vi "ConfigureChannels.vi"(6 "supported metrics":string[](array[string]), 7 "high rate":bool, 8 "error in (no error)":errorcluster, 9 "metric cache":variant, 10 "group":T1, 11 "device":T10) -> (0 "error out":errorcluster, 2 "valid config":bool, 3 "channels":T6[](array[typedef]))   [LabVIEW 2017, in "AnalysisHelper.lvlib"]
uses:
  <vilib>/addons/InsightCM/Utilities/Analysis/Shared/AnalysisHelper.lvlib
  <vilib>/addons/InsightCM/MessageBus/Base/controls/R2_DeviceModel.ctl
  <vilib>/addons/InsightCM/MessageBus/Base/controls/R2_Device.ctl
  <vilib>/addons/InsightCM/MessageBus/Base/controls/KeyValuePair.ctl
  <vilib>/addons/InsightCM/MessageBus/Base/controls/DeviceState.ctl
  <vilib>/addons/InsightCM/MessageBus/Base/controls/R2_DataGroup.ctl
  <vilib>/addons/InsightCM/MessageBus/Base/controls/OperatingState.ctl
  <vilib>/addons/InsightCM/MessageBus/Base/controls/Trigger.ctl
  <vilib>/addons/InsightCM/MessageBus/Base/controls/Condition.ctl
  <vilib>/addons/InsightCM/MessageBus/Base/controls/BurstModeTrigger.ctl
  <vilib>/addons/InsightCM/MessageBus/Base/controls/DeviceSensorGroup.ctl
  <vilib>/addons/InsightCM/MessageBus/Base/controls/WirelessEndpoint.ctl
  <vilib>/addons/InsightCM/MessageBus/Base/controls/WirelessChannel.ctl
  <vilib>/addons/InsightCM/MessageBus/Base/controls/R2_Channel.ctl
  <vilib>/addons/InsightCM/MessageBus/Base/controls/Metric.ctl
  <vilib>/addons/InsightCM/MessageBus/Base/controls/Tag.ctl
  <vilib>/addons/InsightCM/Utilities/Analysis/Shared/controls/Channel.ctl
  <vilib>/addons/InsightCM/Utilities/Analysis/Shared/controls/SpeedType.ctl
  <vilib>/addons/InsightCM/Utilities/Analysis/Shared/controls/Feature.ctl
  <vilib>/addons/InsightCM/Utilities/Analysis/Shared/controls/AmplitudeScale.ctl
  <vilib>/addons/InsightCM/Utilities/Analysis/Shared/controls/SpeedCacheOps.ctl
  <vilib>/addons/InsightCM/Utilities/DeviceModelHelpers/DeviceModelHelpers.lvlib
  <vilib>/addons/InsightCM/Utilities/PropertyHelpers/PropertyHelpers.lvlib
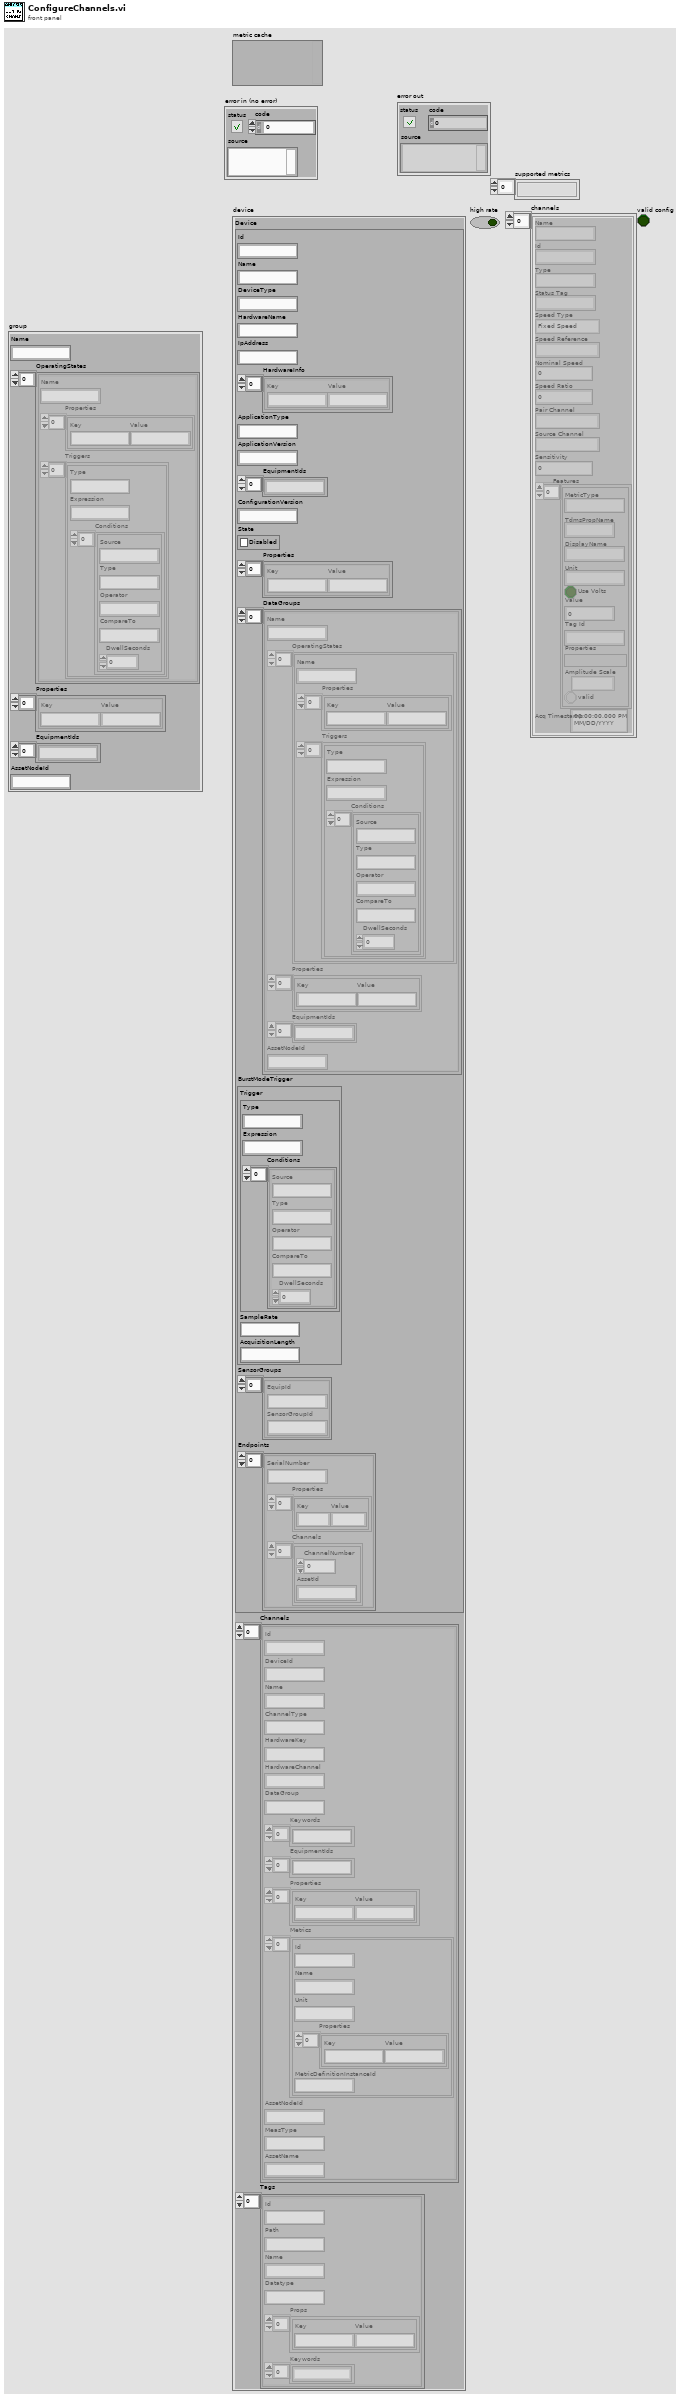
[diagram p1: front panel]
types:
  T1 = typedef "R2_DataGroup.ctl" = cluster{"Name":string, "OperatingStates":T2[], "Properties":T3[], "EquipmentIds":string[], "AssetNodeId":string}
  T2 = typedef "OperatingState.ctl" = cluster{"Name":string, "Properties":T3[], "Triggers":T4[]}
  T3 = typedef "KeyValuePair.ctl" = cluster{"Key":string, "Value":string}
  T4 = typedef "Trigger.ctl" = cluster{"Type":string, "Expression":string, "Conditions":T5[]}
  T5 = typedef "Condition.ctl" = cluster{"Source":string, "Type":string, "Operator":string, "CompareTo":string, "DwellSeconds":dbl}
  T6 = typedef "AnalysisHelper.lvlib/Channel.ctl" = cluster{"Name":string, "Id":string, "Type":string, "Status Tag":string, "Speed Type":T7, "Speed Reference":string, "Nominal Speed":dbl, "Speed Ratio":dbl, "Pair Channel":string, "Source Channel":string, "Sensitivity":dbl, "Features":T8[], "Acq Timestamp":timestamp}
  T7 = typedef "AnalysisHelper.lvlib/SpeedType.ctl" = enum16{"Fixed Speed", "Tachometer", "From Map"}
  T8 = typedef "AnalysisHelper.lvlib/Feature.ctl" = cluster{"MetricType":string, "TdmsPropName":string, "DisplayName":string, "Unit":string, "Use Volts":bool, "Value":dbl, "Tag Id":string, "Properties":variant, "Amplitude Scale":T9, "valid":bool}
  T9 = typedef "AnalysisHelper.lvlib/AmplitudeScale.ctl" = enum16{"rms", "peak", "pk-pk"}
  T10 = typedef "R2_DeviceModel.ctl" = cluster{"Device":T11, "Channels":T17[], "Tags":T19[]}
  T11 = typedef "R2_Device.ctl" = cluster{"Id":string, "Name":string, "DeviceType":string, "HardwareName":string, "IpAddress":string, "HardwareInfo":T3[], "ApplicationType":string, "ApplicationVersion":string, "EquipmentIds":string[], "ConfigurationVersion":string, "State":T12, "Properties":T3[], "DataGroups":T1[], "BurstModeTrigger":T13, "SensorGroups":T14[], "Endpoints":T15[]}
  T12 = typedef "DeviceState.ctl" = cluster{"Disabled":bool}
  T13 = typedef "BurstModeTrigger.ctl" = cluster{"Trigger":T4, "SampleRate":string, "AcquisitionLength":string}
  T14 = typedef "DeviceSensorGroup.ctl" = cluster{"EquipId":string, "SensorGroupId":string}
  T15 = typedef "WirelessEndpoint.ctl" = cluster{"SerialNumber":string, "Properties":T3[], "Channels":T16[]}
  T16 = typedef "WirelessChannel.ctl" = cluster{"ChannelNumber":i32, "AssetId":string}
  T17 = typedef "R2_Channel.ctl" = cluster{"Id":string, "DeviceId":string, "Name":string, "ChannelType":string, "HardwareKey":string, "HardwareChannel":string, "DataGroup":string, "Keywords":string[], "EquipmentIds":string[], "Properties":T3[], "Metrics":T18[], "AssetNodeId":string, "MeasType":string, "AssetName":string}
  T18 = typedef "Metric.ctl" = cluster{"Id":string, "Name":string, "Unit":string, "Properties":T3[], "MetricDefinitionInstanceId":string}
  T19 = typedef "Tag.ctl" = cluster{"Id":string, "Path":string, "Name":string, "Datatype":string, "Props":T3[], "Keywords":string[]}
  T20 = typedef "AnalysisHelper.lvlib/SpeedCacheOps.ctl" = enum16{"Init", "GetSpeed"}
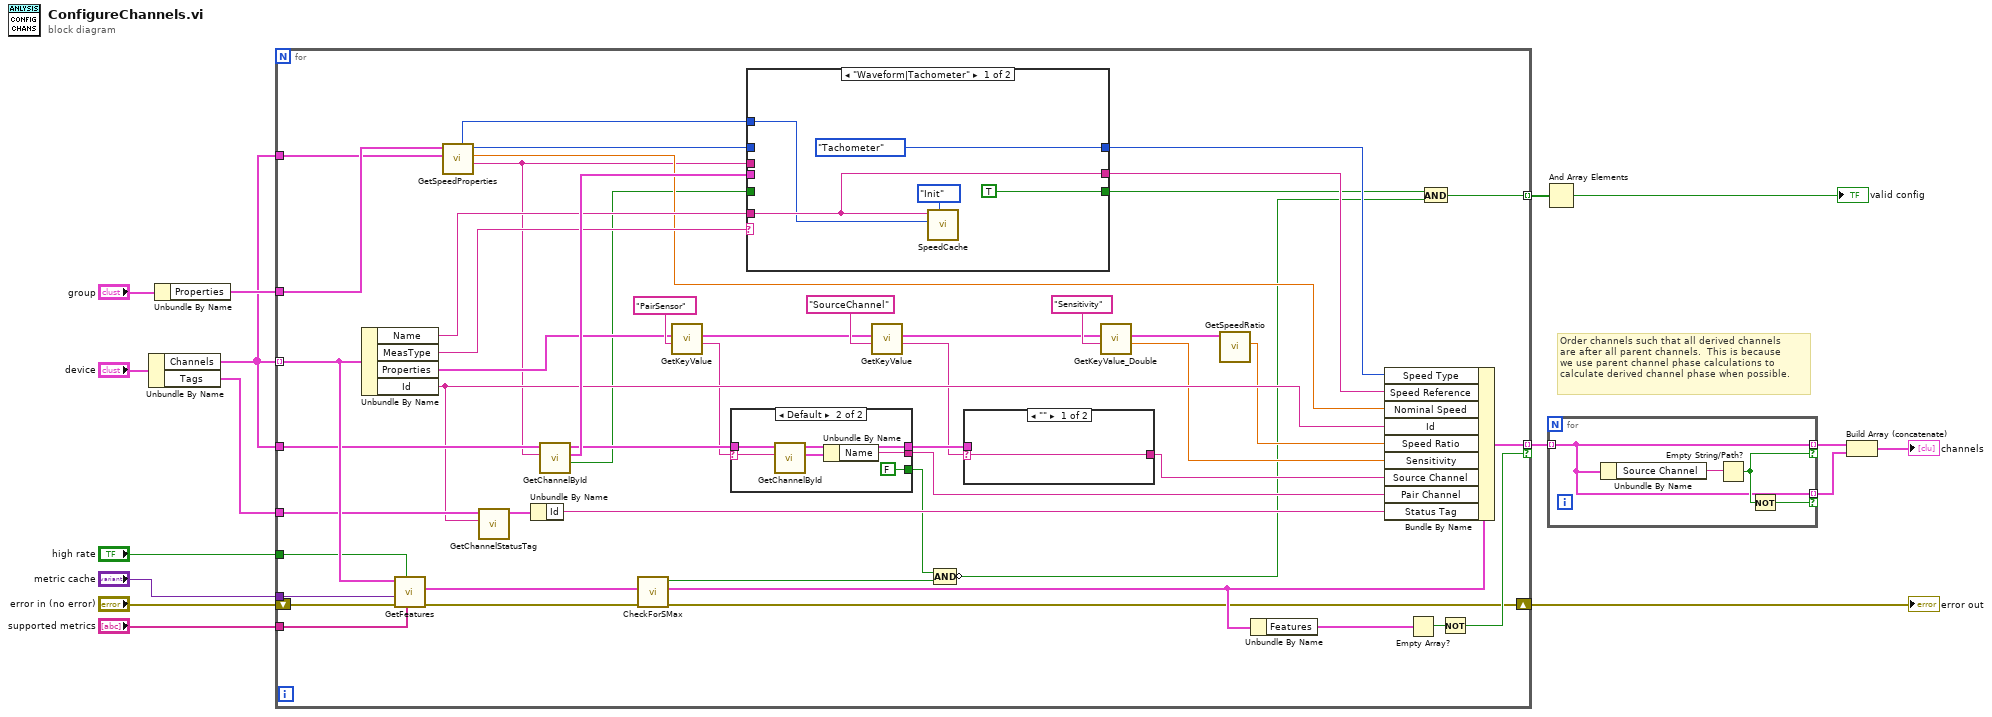
[diagram p0: block diagram]
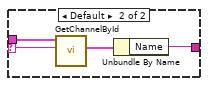
[diagram p2: hidden frame]
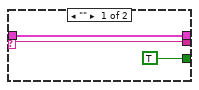
[diagram p3: hidden frame]
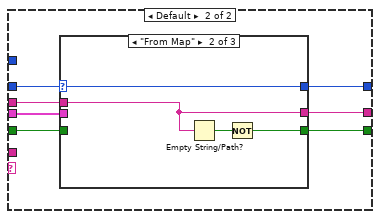
[diagram p4: hidden frame]
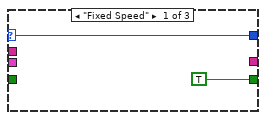
[diagram p5: hidden frame]
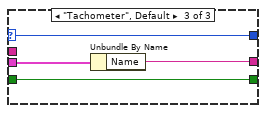
[diagram p6: hidden frame]
diagram:
  # "Order channels such that all derived channels\nare after all parent channels.  This is because\nwe use parent channel phase calculations to\ncalculate derived channel phase when possible."
  n1 = Unbundle By Name("device") -> ("Channels"=w1:T17[], "Tags"=w13:T19[])
  n2 = Unbundle By Name("group") -> ("Properties"=w11:T3[])
  n3 = for {
    tunnel: [w63] -> w9 mode=indexing if=w45
    tunnel: "metric cache" -> [w65]
    tunnel: w1 -> [w64] mode=indexing
    tunnel: w13 -> [w51]
    shift-right: [w27] -> w10
    shift-left: "error in (no error)" -> [w66]
    tunnel: w1 -> [w60]
    tunnel: w11 -> [w42]
    tunnel: "supported metrics" -> [w48]
    tunnel: "high rate" -> [w30]
    tunnel: [w21] -> w3 mode=indexing
    tunnel: w1 -> [w18]
    n4 = Unbundle By Name(w64) -> ("Name"=w58:string, "MeasType"=w57:string, "Properties"=w40:T3[], "Id"=w43:string)
    n5 = call <vilib>:"GetFeatures.vi"("supported metrics"=w48, "high rate"=w30, "error in (no error)"=w66, "Metric Cache"=w65, "ChannelModel"=w64) -> ("error out"=w28:errorcluster, "Chanel"=w26:T6)  [unwired: 5 in]
    n6 = call <vilib>:"GetSpeedProperties.vi"("Channels"=w18, "properties"=w42) -> ("speed reference id"=w19:string, "nominal speed"=w41:dbl, "speed type"=w39:T7, "max empty blocks"=w17:i32)  [unwired: 6 in]
    n7 = call <vilib>:"GetChannelStatusTag.vi"("channel id"=w43, "tags"=w51) -> ("channel status tag"=w50:T19)  [unwired: 9 in]
    n8 = Unbundle By Name(w50) -> ("Id"=w49:string)
    n9 = call <vilib>:"GetChannelById.vi"("channel id"=w19, "channels in"=w60) -> ("found"=w23:bool, "channel"=w62:T17, "channels out"=w61:T17[])  [unwired: 7 in]
    n10 = call <vilib>:"CheckForSMax.vi"("error in (no error)"=w28, "chanel in"=w26) -> ("error out"=w27:errorcluster, "chanel out"=w29:T6, "contains smax"=w25:bool)  [unwired: 7 in]
    n11 = call <vilib>:"GetKeyValue.vi"("key"="PairSensor", "key value pairs"=w40) -> ("value"=w36:string, "key value pairs out"=w44:T3[])  [unwired: 7 in, 1 out]
    n12 = case shown="Default" w36 {
      selector: w36 -> [w73 w76]
      tunnel: w61 -> [w74 w79]
      tunnel: [w73 w78] -> w59
      tunnel: [w74 w77] -> w52
      tunnel: [TRUE FALSE] -> w24
      frame "" {
      }
      frame Default {
        n13 = call <vilib>:"GetChannelById.vi"("channel id"=w76, "channels in"=w79) -> ("channel"=w80:T17, "channels out"=w77:T17[])  [unwired: 7 in, 1 out]
        n14 = Unbundle By Name(w80) -> ("Name"=w78:string)
      }
    }
    n15 = case shown="\"Waveform|Tachometer\"" w57 {
      tunnel: w62 -> [_ w92]
      tunnel: w58 -> [w84 _]
      tunnel: [w84 w91] -> w38
      tunnel: [SpeedType."Tachometer" ("speed type") w89] -> w37
      tunnel: w39 -> [_ w90]
      tunnel: w23 -> [_ w88]
      tunnel: [TRUE ("found") w87] -> w20
      tunnel: w19 -> [_ w86]
      tunnel: w17 -> [w81 _]
      frame "Waveform|Tachometer" {
        n16 = call <vilib>:"SpeedCache.vi"("operation"=SpeedCacheOps."Init", "max empty blocks"=w81, "channel"=w84) -> ()  [unwired: 6 in, 3 out]
      }
      frame Default {
        n17 = case shown="\"From Map\"" w90 {
          selector: w90 -> [w94 w98 w100]
          tunnel: w92 -> [_ _ w102]
          tunnel: [_ w97 w101] -> w91
          tunnel: [w94 w98 w100] -> w89
          tunnel: w88 -> [_ _ w99]
          tunnel: [TRUE ("found") w95 w99] -> w87
          tunnel: w86 -> [_ w97 _]
          frame "Fixed Speed" {
          }
          frame "From Map" {
            n18 = Empty String/Path?(string/path=w97) -> (empty?=w96:bool)
            n19 = Not(x=w96) -> (.not. x?=w95:bool)
          }
          frame "Tachometer", Default {
            n20 = Unbundle By Name(w102) -> ("Name"=w101:string)
          }
        }
      }
    }
    n21 = call <vilib>:"GetKeyValue.vi"("key"="SourceChannel", "key value pairs"=w44) -> ("value"=w35:string, "key value pairs out"=w34:T3[])  [unwired: 7 in, 1 out]
    n22 = Compound Arithmetic op=AND(w24, w25) -> (invert w22:bool)
    n23 = case shown="\"\"" w35 {
      selector: w35 -> [w67 w68]
      tunnel: [w67 w70] -> w53
      tunnel: w52 -> [_ w69]
      frame "" {
      }
      frame Default {
        n24 = call <vilib>:"GetChannelById.vi"("channel id"=w68, "channels in"=w69) -> ("channel"=w71:T17)  [unwired: 7 in, 2 out]
        n25 = Unbundle By Name(w71) -> ("Name"=w70:string)
      }
    }
    n26 = call <vilib>:"GetKeyValue_Double.vi"("key"="Sensitivity" ("Name"), "key value pairs"=w34) -> ("value"=w33:dbl, "key value pairs out"=w32:T3[])  [unwired: 7 in, 1 out]
    n27 = call <vilib>:"GetSpeedRatio.vi"("key value pairs in"=w32) -> ("speed ratio"=w31:dbl)  [unwired: 9 in, 1 out]
    n28 = Unbundle By Name(w29) -> ("Features"=w47:T8[])
    n29 = Bundle By Name(cluster=w29, "Speed Type"=w37, "Speed Reference"=w38, "Nominal Speed"=w41, "Id"=w43, "Speed Ratio"=w31, "Sensitivity"=w33, "Source Channel"=w53, "Pair Channel"=w59, "Status Tag"=w49) -> (w63:T6)
    n30 = Empty Array?(array=w47) -> (empty?=w46:bool)
    n31 = And(x=w20, y=w22) -> (x .and. y?=w21:bool)
    n32 = Not(x=w46) -> (.not. x?=w45:bool)
  }
  "error out" <- w10
  n33 = And Array Elements(Boolean array=w3) -> (logical AND=→"valid config":bool)
  n34 = for {
    tunnel: w9 -> [w104] mode=indexing
    tunnel: [w104] -> w8 mode=indexing if=w105
    tunnel: [w104] -> w7 mode=indexing if=w103
    n35 = Unbundle By Name(w104) -> ("Source Channel"=w106:string)
    n36 = Empty String/Path?(string/path=w106) -> (empty?=w105:bool)
    n37 = Not(x=w105) -> (.not. x?=w103:bool)
  }
  n38 = Build Array (concatenate)(w8, w7) -> (→"channels":T6[])
